vi "AverageAndLog.vi"(5 "error in (no error)":errorcluster) -> (19 "error out":errorcluster)   [LabVIEW 2014, in "IndoorData.lvclass"]
uses:
  IndoorData.lvclass
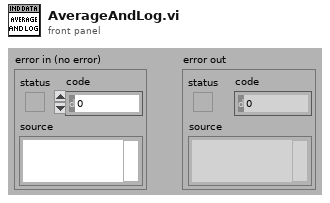
[diagram p1: front panel]
types:
  T1 = enum16{"open", "replace", "create", "open or create", "replace or create", "replace or create with confirmation"}
  T2 = typedef "IndoorData.lvclass/ObjectAttributes.ctl" = cluster{"DebugData":T3, "Actual":T4, "BufferedReadings":T5, "AVGReadings":T5, "DataFolder":path, "FirstLog?":bool}
  T3 = typedef "IndoorData.lvclass/DebugData.ctl" = cluster{"Rev":string, "Location":string, "LoopIdx":i32, "PiCoreTemp":dbl, "Error":errorcluster}
  T4 = typedef "IndoorData.lvclass/ActualValues.ctl" = cluster{"Time":dbl, "Temp":dbl, "RH":dbl}
  T5 = typedef "IndoorData.lvclass/BufferedReadings.ctl" = cluster{"Time":dbl[], "Temp":dbl[], "RH":dbl[]}
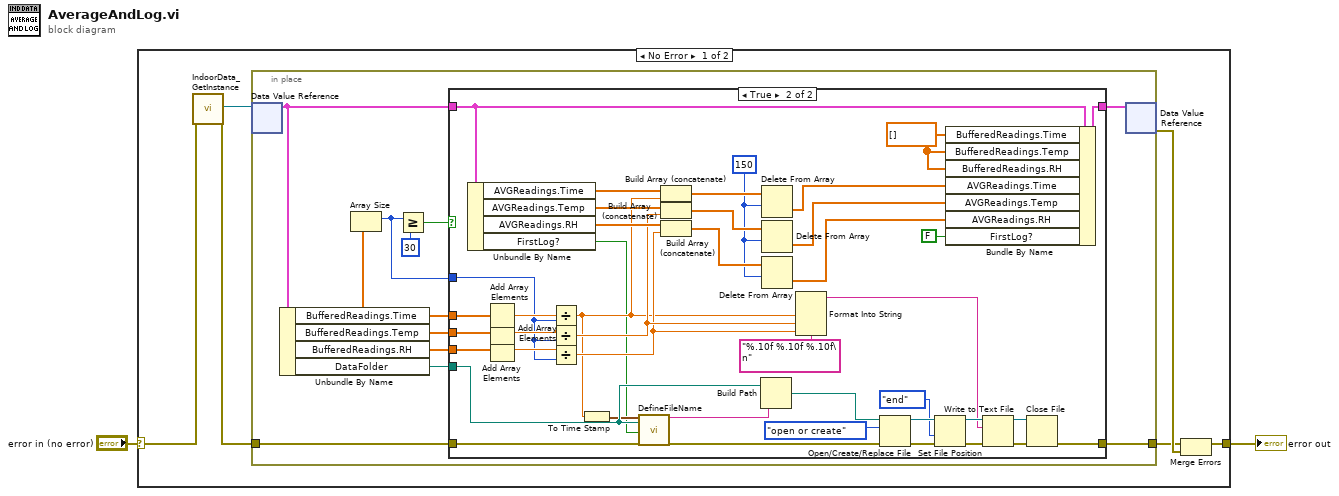
[diagram p0: block diagram]
diagram:
  n1 = case shown="No Error" "error in (no error)" {
    selector: "error in (no error)" -> [w4 w64]
    tunnel: [w3 w64] -> w1
    frame No Error {
      n2 = call "IndoorData_GetInstance.vi"("error in (no error)"=w4) -> ("DVRRefOut"=w7:refnum<data-value>, "error out"=w6:errorcluster)  [unwired: 14 in, 3 out]
      n3 = in-place {
        in-place-border: w6 -> [w14]
        in-place-border: [w15] -> w5
        n4 = in-place-dvr #1(w7) -> (w18:T2)  [unwired: 1 out]
        n5 = Unbundle By Name(w18) -> ("BufferedReadings.Time"=w13:dbl[], "BufferedReadings.Temp"=w12:dbl[], "BufferedReadings.RH"=w11:dbl[], "DataFolder"=w9:path)
        n6 = Array Size(array=w13) -> (size(s)=w10:i32)
        n7 = Greater Or Equal?(x=w10, y=30) -> (x >= y?=w16:bool)
        n8 = case shown="True" w16 {
          tunnel: [w21 w63] -> w19
          tunnel: w18 -> [w21 w54]
          tunnel: [w20 w29] -> w15
          tunnel: w14 -> [w20 w40]
          tunnel: w13 -> [_ w62]
          tunnel: w12 -> [_ w61]
          tunnel: w11 -> [_ w60]
          tunnel: w10 -> [_ w56]
          tunnel: w9 -> [_ w26]
          frame False {
          }
          frame True {
            w47 = 150 ("length")
            w55 = dbl[] [] ("BufferedReadings.Time")
            n9 = Unbundle By Name(w54) -> ("AVGReadings.Time"=w53:dbl[], "AVGReadings.Temp"=w52:dbl[], "AVGReadings.RH"=w51:dbl[], "FirstLog?"=w22:bool)
            n10 = Add Array Elements(numeric array=w62) -> (sum=w59:dbl)
            n11 = Add Array Elements(numeric array=w61) -> (sum=w58:dbl)
            n12 = Add Array Elements(numeric array=w60) -> (sum=w57:dbl)
            n13 = Divide(x=w59, y=w56) -> (x/y=w25:dbl)
            n14 = Divide(x=w58, y=w56) -> (x/y=w42:dbl)
            n15 = Divide(x=w57, y=w56) -> (x/y=w41:dbl)
            n16 = To Time Stamp(1:w25) -> (0:w24:timestamp)
            n17 = call "DefineFileName.vi"("Sample Time"=w24, "DataFolder"=w26, "FirstLog?"=w22, "error in (no error)"=w40) -> ("FileName"=w27:string, "error out"=w30:errorcluster)  [unwired: 14 in]
            n18 = Build Array (concatenate)(w53, w25) -> (w50:dbl[])
            n19 = Build Array (concatenate)(w52, w42) -> (w49:dbl[])
            n20 = Build Array (concatenate)(w51, w41) -> (w48:dbl[])
            n21 = Build Path(base path=w26, name or relative path=w27) -> (appended path=w31:path)
            n22 = Delete From Array(array=w50, length=w47) -> (deleted portion=w44:dbl[])  [unwired: 1 in, 1 out]
            n23 = Delete From Array(array=w49, length=w47) -> (deleted portion=w45:dbl[])  [unwired: 1 in, 1 out]
            n24 = Delete From Array(array=w48, length=w47) -> (deleted portion=w46:dbl[])  [unwired: 1 in, 1 out]
            n25 = Format Into String(format string="%.10f %.10f %.10f\n", w25, w42, w41) -> (resulting string=w28:string)  [unwired: 2 in, 1 out]
            n26 = Open/Create/Replace File(file path (use dialog)=w31, error in=w30, operation (0:open)=T1."open or create") -> (refnum out=w38:refnum<file>, error out=w37:errorcluster)  [unwired: 3 in, 1 out]
            n27 = Set File Position(refnum=w38, from (0:start)=enum16{"start", "end", "current"}."end", error in=w37) -> (refnum out=w34:refnum<file>, error out=w35:errorcluster)  [unwired: 1 in]
            n28 = Bundle By Name(cluster=w54, "BufferedReadings.Time"=w55, "BufferedReadings.Temp"=w55, "BufferedReadings.RH"=w55, "AVGReadings.Time"=w44, "AVGReadings.Temp"=w45, "AVGReadings.RH"=w46, "FirstLog?"=FALSE ("Reboot?")) -> (w63:T2)
            n29 = Write to Text File(file (use dialog)=w34, text=w28, error in=w35) -> (refnum out=w33:refnum<file>, error out=w32:errorcluster)  [unwired: 1 in, 1 out]
            n30 = Close File(refnum=w33, error in=w32) -> (error out=w29:errorcluster)  [unwired: 1 out]
          }
        }
        n31 = in-place-dvr #1(w19) -> (w8:errorcluster)  [unwired: 1 out]
      }
      n32 = Merge Errors(w5, w8) -> (w3:errorcluster)
    }
    frame Error {
    }
  }
  "error out" <- w1
